vi "Read-Sequence.vi"(0 "error in (no error)":errorcluster, 3 "VISA Refnum in":refnum<visa-resource-name>, 7 "Num de tramas":i32, 9 "Tamaño Script":i32, 10 "TRANSDUCTORES":u16) -> (2 "Raw data":T1(array[cluster]), 8 "error out":errorcluster, 11 "VISA reference":refnum<visa-resource-name>)   [LabVIEW 2014, in "CAP-USB.lvlib"]
uses:
  CAP-USB.lvlib
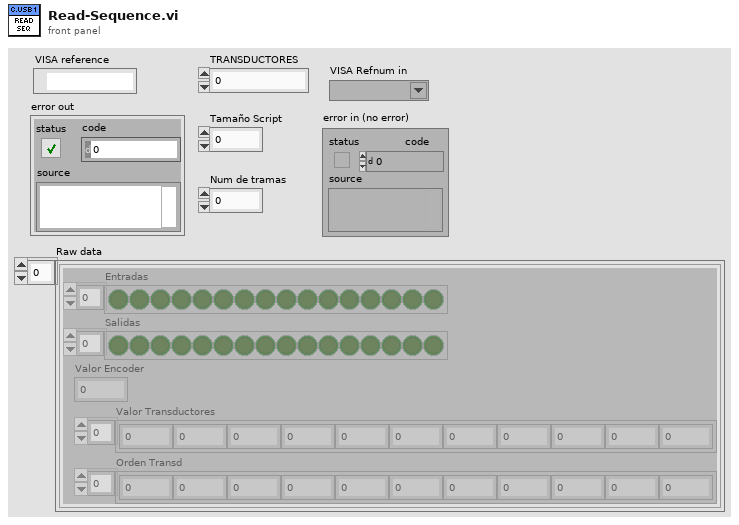
[diagram p1: front panel]
types:
  T1 = cluster{"Entradas":bool[], "Salidas":bool[], "Valor Encoder":u16, "Valor Transductores":u16[], "Orden Transd":i32[]}[]
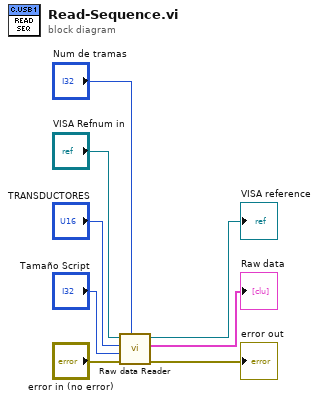
[diagram p0: block diagram]
diagram:
  n1 = call "Raw data Reader.vi"("Num de tramas"="Num de tramas", "error in (no error)"="error in (no error)", "Tamaño Script"="Tamaño Script", "TRANSDUCTORES"="TRANSDUCTORES", "VISA Refnum in"="VISA Refnum in") -> ("error out"=→"error out":errorcluster, "Raw data"=→"Raw data":T1, "VISA reference"=→"VISA reference":refnum<visa-resource-name>)  [unwired: 2 in]
